vi "BasicExampleWithInstrFrwk.vi"() -> ()   [LabVIEW 2015]
uses:
  <vilib>/Platform/TimedLoop/XDataNode/wakeup.ctl
  <vilib>/Platform/TimedLoop/XDataNode/XDNodeRunTimeDep.lvlib
  <vilib>/Platform/TimedLoop/XDataNode/nitl_modes.ctl
  <vilib>/Platform/TimedLoop/XDataNode/timing_clust.ctl
  <vilib>/Platform/TimedLoop/XDataNode/XDataNode.xnode
  <instrlib>/_niInstr/Instruction Framework/v1/FPGA/Top Level Bus/Register Configuration/Register Configuration.lvclass
  <vilib>/eio/EIONode/EIONode.xnode
  Core/ScaleAndLimit.lvlib
  Core/AddressSpace.lvclass
  <vilib>/rvi/eio/common/nirviEmuTemplateMethod_errors.vi
  <instrlib>/_niInstr/FIFO Register Bus/v1/FPGA/niInstr FIFO Register Bus v1 FPGA.lvclass
panel:
  in  "fifo reg bus ctrl 0":u32
  out "fifo reg bus status 0":u32
  out "fifo reg bus data 0":u64
  in  "DummyChannel15":i16
  out "SimultaneousAILoopRate":u32
  out "ScaledAI":sgl[](array[numeric])
  # "Device Utilization\n---------------------------\nTotal Slices: 37.8% (5026 out of 13300)\nSlice Registers: 13.6% (14426 out of 106400)\nSlice LUTs: 24.6% (13113 out of 53200)\nBlock RAMs: 2.9% (4 out of 140)\nDSP48s: 1.4% (3 out of 220)"
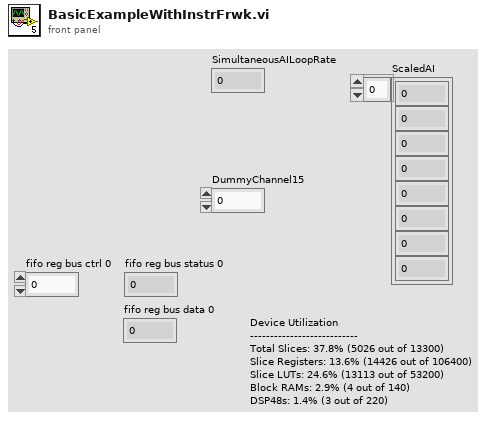
[diagram p1: front panel]
types:
  T1 = typedef "XDNodeRunTimeDep.lvlib/timing_clust.ctl" = cluster{"Expected End [f-1]":u64, "Actual End [f-1]":u64, "Finished Late? [f-1]":bool, "Expected End [i-1]":u64, "Actual End [i-1]":u64, "Finished Late? [i-1]":bool, "Expected Start [i]":u64, "Actual Start [i]":u64, "Expected Start [f]":u64, "Actual Start [f]":u64, "Source Name":string, "Structure Name":string, "Period":i64, "Deadline":i64, "Offset":i64, "Start":i64, "Priority":i32, "Timeout":i32, "Mode":T2, "Wakeup Reason":T3, "Error":errorcluster, "Source Type":string, "Secondary Source Type":string, "Global End Time":u64, "Global Start Time":u64, "Frame Duration":u64, "Iteration Duration":u64, "Assigned CPU":i32, "I/O Scan Engine Mode":u32}
  T2 = typedef "XDNodeRunTimeDep.lvlib/nitl_modes.ctl" = enum32{"No Change", "Process missed periods, maintain original phase", "Discard missed periods, maintain original phase", "Process missed periods, ignore original phase", "Discard missed periods, ignore original phase"}
  T3 = typedef "XDNodeRunTimeDep.lvlib/wakeup.ctl" = enum32{"Normal", "Aborted", "Asynchronous wakeup", "Timing source error", "Timed loop error", "Timeout"}
  T4 = typedef "ScaleAndLimit.lvlib/LimitsRegisters.ctl" = cluster{"HighLimits":refnum<k21>, "LowLimits":refnum<k21>, "ClearLimits":refnum<k21>, "LimitsFlag":refnum<k21>}
  T5 = typedef "ScaleAndLimit.lvlib/ConfigRegisters.ctl" = cluster{"LimitsEnabled":refnum<k21>, "UnscaledHighLimit":refnum<k21>, "UnscaledLowLimit":refnum<k21>, "B":refnum<k21>, "M":refnum<k21>}
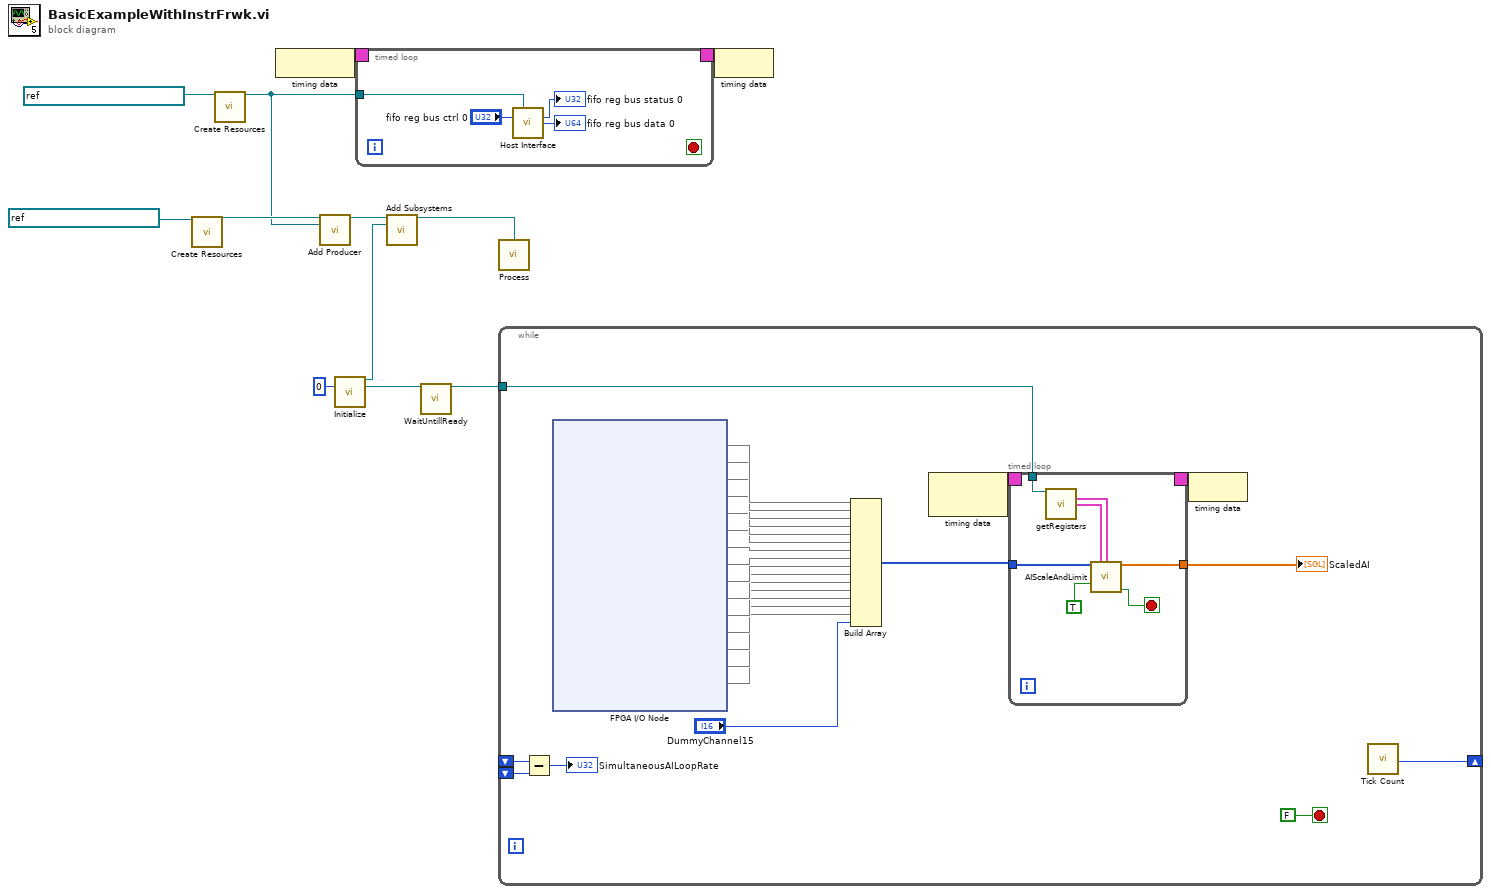
[diagram p0: block diagram]
diagram:
  n1 = call <instrlib>:"Create Resources.vi"("register clock"=refnum<k21> "40 MHz Onboard Clock") -> ("register configuration"=w12:refnum<class "Register Configuration.lvclass">)  [unwired: 14 in]
  n2 = call <instrlib>:"Create Resources.vi"("instruction fifo"=refnum<k21> "reg.host instruction fifo 0") -> ("fifo register bus"=w1:refnum<class "niInstr FIFO Register Bus v1 FPGA.lvclass">)  [unwired: 14 in]
  n3 = node-c288() -> (w4:T1)
  n4 = call <instrlib>:"Add Producer.vi"("register configuration in"=w12, "instruction producer"=w1) -> ("register configuration out"=w10:refnum<class "Register Configuration.lvclass">)  [unwired: 13 in]
  n5 = call "Initialize.vi"("instance"=u8 0) -> ("subsystem"=w9:refnum<class "Single Address Space Collection.lvclass">, "AddressSpace"=w6:refnum<class "AddressSpace.lvclass">)  [unwired: 13 in]
  n6 = timed-loop {
    timing: w4 -> [_]
    timing-out: [_] -> w3
    tunnel: w1 -> [w16]
    stop <- _ stop-if-true
    n7 = call <instrlib>:"Host Interface.vi"("fifo register bus"=w16, "fifo reg bus ctrl 0"="fifo reg bus ctrl 0") -> ("fifo reg bus status 0"=→"fifo reg bus status 0":u32, "fifo reg bus data 0"=→"fifo reg bus data 0":u64)  [unwired: 12 in]
  }
  n8 = call <instrlib>:"Add Subsystems.vi"("register configuration in"=w10, "subsystems"=w9) -> ("register configuration out"=w7:refnum<class "Register Configuration.lvclass">)  [unwired: 13 in]
  n9 = call "WaitUntillReady.vi"("AddressSpace in"=w6) -> ("AddressSpace out"=w5:refnum<class "AddressSpace.lvclass">)  [unwired: 14 in]
  n10 = call <instrlib>:"Process.vi"("register configuration"=w7) -> ()  [unwired: 15 in]
  n11 = while {
    shift-right: [w43] -> _
    shift-left: _ -> [w42]
    shift-left: _ -> [w41]
    tunnel: w5 -> [w21]
    stop <- FALSE stop-if-true
    n12 = Subtract(x=w42, y=w41) -> (x-y=→"SimultaneousAILoopRate":u32)
    n13 = xnode "FPGA I/O Node"() -> ("RMC/Simultaneous/AI0"=w39, "RMC/Simultaneous/AI1"=w38, "RMC/Simultaneous/AI2"=w37, "RMC/Simultaneous/AI3"=w36, "RMC/Simultaneous/AI4"=w35, "RMC/Simultaneous/AI5"=w34, "RMC/Simultaneous/AI6"=w33, "RMC/Simultaneous/AI7"=w32, "RMC/Simultaneous/AI8"=w31, "RMC/Simultaneous/AI9"=w30, "RMC/Simultaneous/AI10"=w29, "RMC/Simultaneous/AI11"=w28, "RMC/Simultaneous/AI12"=w27, "RMC/Simultaneous/AI13"=w26, "RMC/Simultaneous/AI14"=w25)  [unwired: 16 in, 17 out]
    n14 = Build Array(w39, w38, w37, w36, w35, w34, w33, w32, w31, w30, w29, w28, w27, w26, w25, "DummyChannel15") -> (w20:i16[])
    n15 = node-c288() -> (w24:T1)  [unwired: 1 in]
    n16 = timed-loop {
      timing: w24 -> [_]
      timing-out: [_] -> w23
      tunnel: w20 -> [w51]
      tunnel: [w49] -> w22
      tunnel: w21 -> [w47]
      stop <- w48 stop-if-true
      n17 = call "getRegisters.vi"("AddressSpace in"=w47) -> ("LimitsRegisters"=w46:T4, "ConfigRegisters"=w45:T5)  [unwired: 12 in, 1 out]
      n18 = call "AIScaleAndLimit.vi"("UnscaledAI"=w51, "ConfigRegisters"=w45, "LimitsRegisters"=w46, "input valid"=TRUE) -> ("ScaledAI"=w49:sgl[], "output valid"=w48:bool)  [unwired: 6 in, 4 out]
    }
    "ScaledAI" <- w22
    n19 = node-c288(w23) -> ()
    n20 = call "Tick Count"() -> ("Tick Count(Ticks)"=w43:u32)
  }
  n21 = node-c288(w3) -> ()
